vi "intersect_triangleCulling.vi"(5 "vert2":dbl[](array[numeric]), 7 "vert1":dbl[](array[numeric]), 8 "vert0":dbl[](array[numeric]), 9 "dir":dbl[](array[numeric]), 10 "orig":dbl[](array[numeric])) -> (0 "v":dbl format="%.2f", 1 "u":dbl format="%.2f", 2 "t":dbl format="%.2f", 3 "intersect":bool)   [LabVIEW 2019]
doc: "This file corresponds to the Code of the IF part (with culling) of the \"Fast, Minimum Storage Ray/Triangle Intersection\" from Tomas Möller and Ben Trumbore\nINPUT: three vertecies of a triangle (vert0, vert1, vert2), the origin (orig) and direction vector (dir) of the lign.\nOUTPUT: bool \"intersect\" indicating the intersection between triangle and lign, barycentric coordinates of the triangle intersection point (u,v) and distance t of the origin to the intersection point.\n\nJean-Claude Metzger, 16.01.2012"
uses:
  <vilib>/Analysis/baseanly.llb/Real Dot Product.vi
  <vilib>/Analysis/NI_AALPro.lvlib
  <vilib>/Analysis/NI_AALBase.lvlib
panel:
  out "inv_det":dbl
  out "qvec":dbl[](array[numeric])
  out "tvec":dbl[](array[numeric])
  out "det":dbl format="%.2f"
  out "pvec":dbl[](array[numeric])
  out "edge2":dbl[](array[numeric])
  out "edge1":dbl[](array[numeric])
  # "This file corresponds to the  Code of the IF part (with culling) of the \"Fast, Minimum Storage Ray/Triangle Intersection\" from Tomas Möller and Ben Trumbore\nINPUT: three vertecies of a triangle (vert0, vert1, vert2), the origin (orig) and direction vector (dir) of the lign.\nOUTPUT: bool \"intersect\" indicating the intersection between triangle and lign, barycentric coordinates of the triangle intersection point (u,v) and distance t of the origin to the intersection point.\n\nJean-Claude Metzger, 16.01.2012"
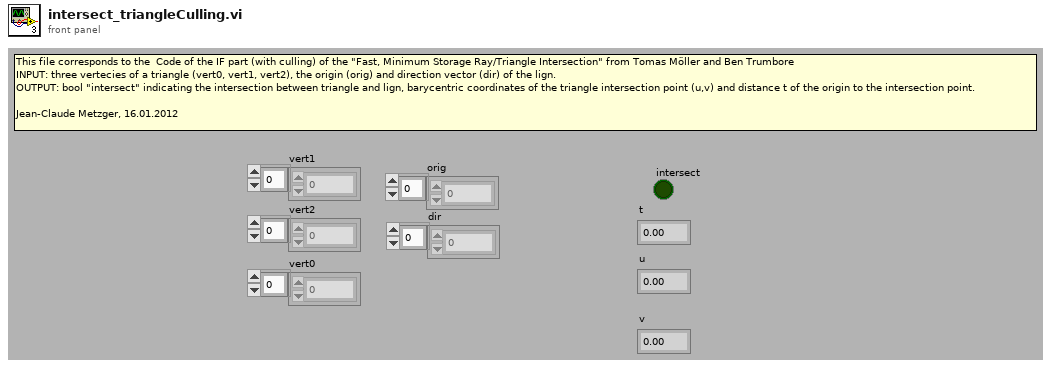
[diagram p1: front panel]
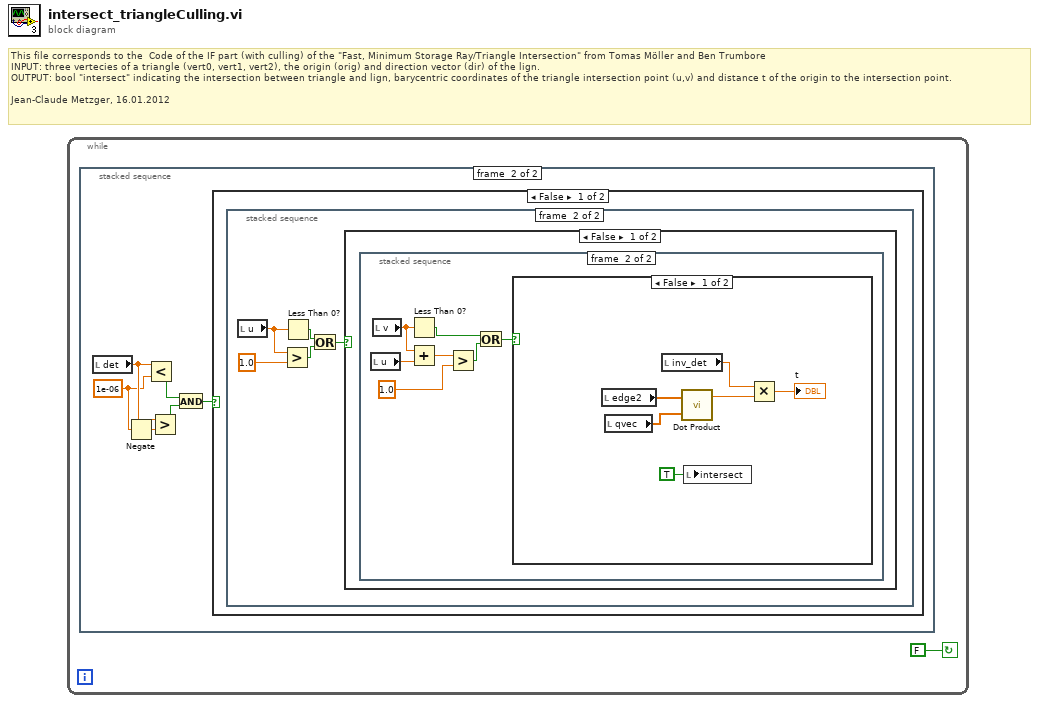
[diagram p0: block diagram]
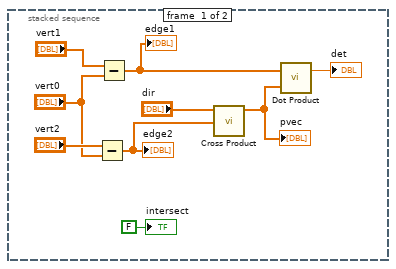
[diagram p2: hidden frame]
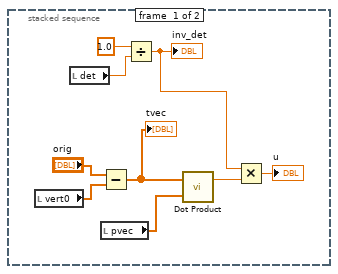
[diagram p3: hidden frame]
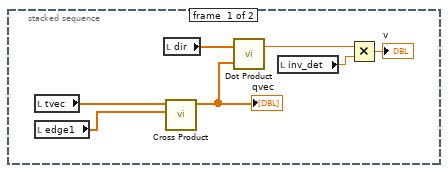
[diagram p4: hidden frame]
diagram:
  # "This file corresponds to the  Code of the IF part (with culling) of the \"Fast, Minimum Storage Ray/Triangle Intersection\" from Tomas Möller and Ben Trumbore\nINPUT: three vertecies of a triangle (vert0, vert1, vert2), the origin (orig) and direction vector (dir) of the lign.\nOUTPUT: bool \"intersect\" indicating the intersection between triangle and lign, barycentric coordinates of the triangle intersection point (u,v) and distance t of the origin to the intersection point.\n\nJean-Claude Metzger, 16.01.2012"
  n1 = while {
    stop <- FALSE continue-if-true
    n2 = stacked-sequence {
      frame #0 {
        n3 = Subtract(x="vert2", y="vert0") -> (x-y=w6:dbl[])
        "edge2" <- w6
        n4 = Subtract(x="vert1", y="vert0") -> (x-y=w4:dbl[])
        "edge1" <- w4
        n5 = call <vilib>:"Cross Product.vi"("B Vector"=w6, "A Vector"="dir") -> ("Cross Product"=w5:dbl[])  [unwired: 8 in, 1 out]
        "pvec" <- w5
        n6 = call-poly <vilib>:"Dot Product.vi"("Y Vector"=w5, "X Vector"=w4) -> ("X * Y"=→"det":dbl)  [unwired: 1 out]
        "intersect" <- FALSE ("intersect")
      }
      frame #1 {
        w12 = 1e-06 ("y")
        n7 = local read "det"() -> (w13:dbl)
        n8 = Negate(x=w12) -> (-x=w11:dbl)
        n9 = Less?(x=w13, y=w12) -> (x < y?=w15:bool)
        n10 = Greater?(x=w13, y=w11) -> (0:w14:bool)
        n11 = And(x=w15, y=w14) -> (x .and. y?=w16:bool)
        n12 = case shown="False" w16 {
          frame False {
            n13 = stacked-sequence {
              frame #0 {
                n14 = local read "vert0"() -> (w24:dbl[])
                n15 = local read "det"() -> (w20:dbl)
                n16 = Subtract(x="orig", y=w24) -> (x-y=w23:dbl[])
                "tvec" <- w23
                n17 = local read "pvec"() -> (w22:dbl[])
                n18 = Divide(x=1.0, y=w20) -> (x/y=w17:dbl)
                "inv_det" <- w17
                n19 = call-poly <vilib>:"Dot Product.vi"("Y Vector"=w22, "X Vector"=w23) -> ("X * Y"=w18:dbl)  [unwired: 1 out]
                n20 = Multiply(x=w17, y=w18) -> (x*y=→"u":dbl)
              }
              frame #1 {
                n21 = local read "u"() -> (w30:dbl)
                n22 = Greater?(x=w30, y=1.0) -> (0:w28:bool)
                n23 = Less Than 0?(x=w30) -> (x < 0?=w29:bool)
                n24 = Or(x=w29, y=w28) -> (x .or. y?=w27:bool)
                n25 = case shown="False" w27 {
                  frame False {
                    n26 = stacked-sequence {
                      frame #0 {
                        n27 = local read "tvec"() -> (w37:dbl[])
                        n28 = local read "edge1"() -> (w36:dbl[])
                        n29 = local read "dir"() -> (w35:dbl[])
                        n30 = call <vilib>:"Cross Product.vi"("B Vector"=w36, "A Vector"=w37) -> ("Cross Product"=w34:dbl[])  [unwired: 8 in, 1 out]
                        "qvec" <- w34
                        n31 = call-poly <vilib>:"Dot Product.vi"("Y Vector"=w34, "X Vector"=w35) -> ("X * Y"=w33:dbl)  [unwired: 1 out]
                        n32 = local read "inv_det"() -> (w31:dbl)
                        n33 = Multiply(x=w33, y=w31) -> (x*y=→"v":dbl)
                      }
                      frame #1 {
                        n34 = local read "u"() -> (w41:dbl)
                        n35 = local read "v"() -> (w42:dbl)
                        n36 = Less Than 0?(x=w42) -> (x < 0?=w43:bool)
                        n37 = Add(x=w42, y=w41) -> (x+y=w40:dbl)
                        n38 = Greater?(x=w40, y=1.0) -> (0:w44:bool)
                        n39 = Or(x=w43, y=w44) -> (x .or. y?=w39:bool)
                        n40 = case shown="False" w39 {
                          frame False {
                            n41 = local read "edge2"() -> (w50:dbl[])
                            n42 = local read "qvec"() -> (w49:dbl[])
                            n43 = local read "inv_det"() -> (w46:dbl)
                            n44 = call-poly <vilib>:"Dot Product.vi"("Y Vector"=w49, "X Vector"=w50) -> ("X * Y"=w47:dbl)  [unwired: 1 out]
                            n45 = local write "intersect"(TRUE ("intersect")) -> ()
                            n46 = Multiply(x=w46, y=w47) -> (x*y=→"t":dbl)
                          }
                          frame True {
                          }
                        }
                      }
                    }
                  }
                  frame True {
                  }
                }
              }
            }
          }
          frame True {
          }
        }
      }
    }
  }
